vi "Test_WriteItem_DeleteItemWithTypeCheck_ItemRemoved.vi"(8 "error in (no error)":errorcluster, 11 "TestCase in":refnum<class "TestComposedLookupTable.lvclass">) -> (0 "error out":errorcluster, 3 "TestCase out":refnum<class "TestComposedLookupTable.lvclass">)   [LabVIEW 2017, in "TestComposedLookupTable.lvclass"]
uses:
  TestComposedLookupTable.lvclass
  Source/LookupTable/LookupTable.lvclass/LookupTable.ctl
  d2ce3032-cee0-48a5-954b-175b0ad98104.vi
  04775304-6477-4e0e-aa98-004dafc2bbf7.vi
  e280f436-a9ad-4fbb-83d7-e5b5a20d87ee.vi
  Source/LookupTable/Read Table Reference.vi
  d2ce3032-cee0-48a5-954b-175b0ad98104.vi/51f8b606-e63b-4647-a103-515e1de43722.vi
  e280f436-a9ad-4fbb-83d7-e5b5a20d87ee.vi/6760c817-0cfb-487c-8443-83d3086cc85e.vi
  Source/LookupTable/LookupTable.lvclass
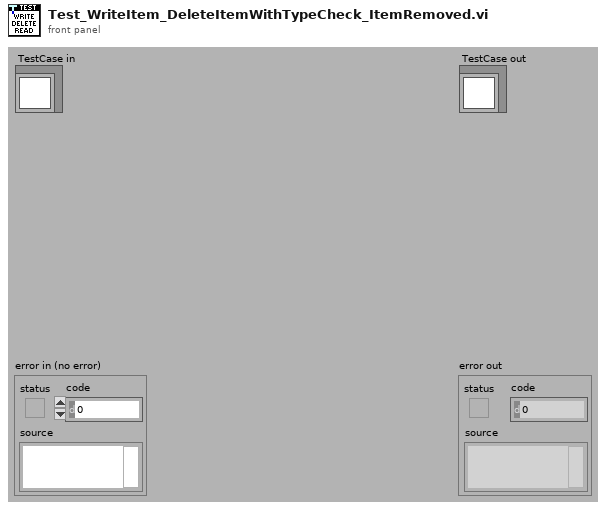
[diagram p1: front panel]
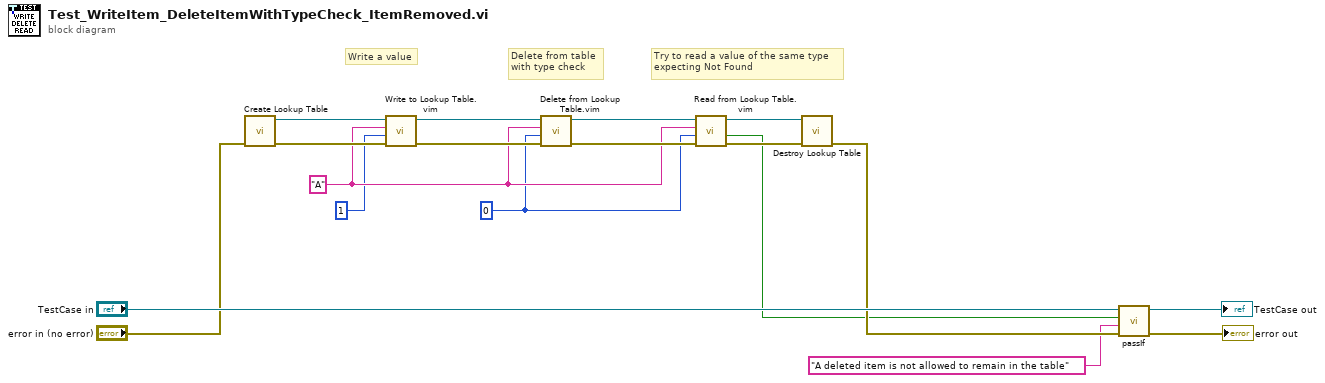
[diagram p0: block diagram]
diagram:
  w2 = 0
  w5 = "A" ("Item Name")
  # "Delete from table\nwith type check"
  # "Try to read a value of the same type\nexpecting Not Found"
  # "Write a value"
  n1 = call "Create Lookup Table.vi"("error in (no error)"="error in (no error)") -> ("error out"=w18:errorcluster, "LookupTable Reference"=w13:refnum<data-value>)  [unwired: 9 in]
  n2 = call "Write to Lookup Table.vim"("error in (no error)"=w18, "Item"=1, "Item Name"=w5, "LookupTable Reference"=w13) -> ("error out"=w17:errorcluster, "LookupTable Reference Out"=w7:refnum<data-value>)  [unwired: 5 in, 1 out]
  n3 = call "Delete from Lookup Table.vim"("error in (no error)"=w17, "Confirm Type"=w2, "Item Name"=w5, "LookupTable Reference"=w7) -> ("error out"=w8:errorcluster, "LookupTable Reference Out"=w6:refnum<data-value>)  [unwired: 5 in, 1 out]
  n4 = call "Read from Lookup Table.vim"("error in (no error)"=w8, "Type"=w2, "Item Name"=w5, "LookupTable Reference"=w6) -> ("error out"=w10:errorcluster, "Not Found?"=w4:bool, "LookupTable Reference Out"=w11:refnum<data-value>)  [unwired: 4 in, 1 out]
  n5 = call "Destroy Lookup Table.vi"("error in (no error)"=w10, "LookupTable Reference"=w11) -> ("error out"=w9:errorcluster)  [unwired: 9 in]
  n6 = call-dynamic "passIf.vi"("error in (no error)"=w9, "message (\"\")"="A deleted item is not allowed to remain in the table" ("message (\"\")"), "pass"=w4, "TestCase in"="TestCase in") -> ("error out"=→"error out":errorcluster, "TestCase out"=→"TestCase out":refnum<class "TestComposedLookupTable.lvclass">)  [unwired: 6 in]
